vi "PolarizationSimulation.vi"() -> ()   [LabVIEW 2020]
uses:
  D:/LabVIEW/Integrated-Neural-Net-master/Integrated-Neural-Net-master (1)/Integrated-Neural-Net-master/Integrated ANN/Sub-VIs/Adam_data.ctl
  <vilib>/Utility/xml.llb/Read From XML File(string).vi
  <vilib>/Utility/xml.llb/Write to XML File(string).vi
  <vilib>/Analysis/NI_AALBase.lvlib
panel:
  in  "Regularization":T1
  in  "Batch Size":i16
  out "NN Loss":dbl(graph)
  in  "Loss Function":enum16{"MSE", "MAE"}(ring)
  in  "Parameters File Path":path
  out "NN Error":dbl
  in  "Training?":bool
  out "NN Output":dbl
  in  "Speed\nMultiplier":dbl=1.0
  in  "AFP On":bool
  in  "AFP Efficiency":dbl=0.9 min=0.0 max=1.0 step=0.01
  in  "AFP Control":cluster{i32, i32}(slide)={200, 230} scale=0.0..500.0
  out "lower R-value AFP":dbl
  out "upper R-value AFP":dbl
  in  "STOP":bool
  in  "Microwave Power":dbl=1.0
  in  "Lower Fit\nParameter":dbl=-3.6
  in  "Upper Fit\nParameter":dbl=3.6
  in  "Std Dev Noise":dbl step=0.0001
  out "lower R-value":dbl
  out "upper R-value":dbl
  in  "RF Control":cluster{i32, i32}(slide)={200, 230} scale=0.0..500.0
  out "p":dbl format="%_4g"
  out "r":dbl
  in  "Saturation\nPolarization":dbl=0.8 min=0.0 max=0.99 step=0.01
  out "Reimann \nsum of Q":dbl format="%_4g"
  out "Corrected Data (Q)":cluster{dbl[], dbl[]}(graph)
  in  "Select Target Type":u16(ring)=2 items=["Test Case", "Deuteron"]
  in  "Reset":bool
  out "Total Polarization (P)":cluster{dbl, dbl}(graph)
  in  "Spin Manipulation\nPower Factor":dbl=0.005
  in  "Decay Spin\nManipulation":bool
  out "Reimann\nsum of P":dbl format="%_4g"
  out "Corrected Data (P)":cluster{dbl[], dbl[]}[](graph)
  out "Signal and Fit (P)":cluster{dbl[], "Best Polynomial Fit":dbl[]}[](graph)
  in  "Positive\nPolarization":bool
  in  "Microwave on":bool
  # "Neural Network"
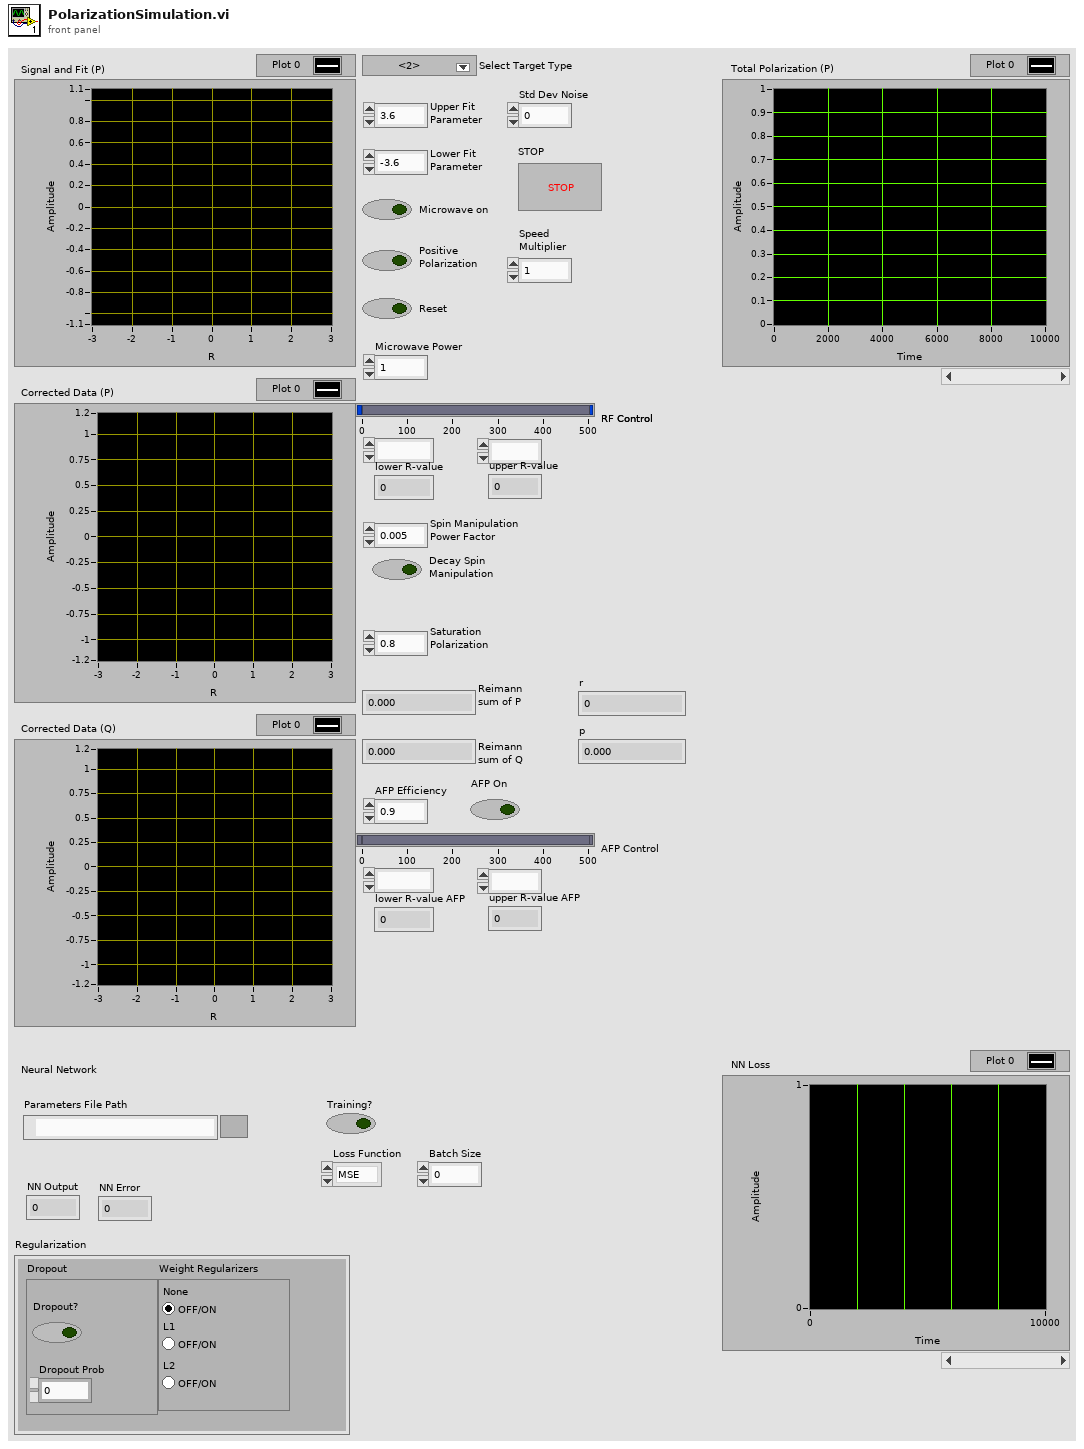
[diagram p1: front panel]
types:
  T1 = cluster{"Dropout":cluster{"Dropout?":bool, "Dropout Prob":dbl}, "Weight Regularizers":enum32{"None", "L1", "L2"}}
  T2 = typedef "Adam_data.ctl" = cluster{"Mw Moments":cluster{"3 ":dbl[], "2":dbl[][], "1":dbl[][]}, "Vw Moments":cluster{"3":dbl[], "2":dbl[][], "1":dbl[][]}, "Mb Moments":cluster{"3":dbl, "2":dbl[], "1":dbl[]}, "Vb Moments":cluster{"3":dbl, "2":dbl[], "1":dbl[]}}
  T3 = cluster{cluster{dbl[][], dbl[]}, cluster{dbl[][], dbl[]}, cluster{dbl[], dbl}}
  T4 = cluster{cluster{"Updated Weights":dbl[][], "Updated Biases":dbl[]}, cluster{"Updated Weights":dbl[][], "Updated Biases":dbl[]}, cluster{"Updated Weights":dbl[], "Updated Biases":dbl}}
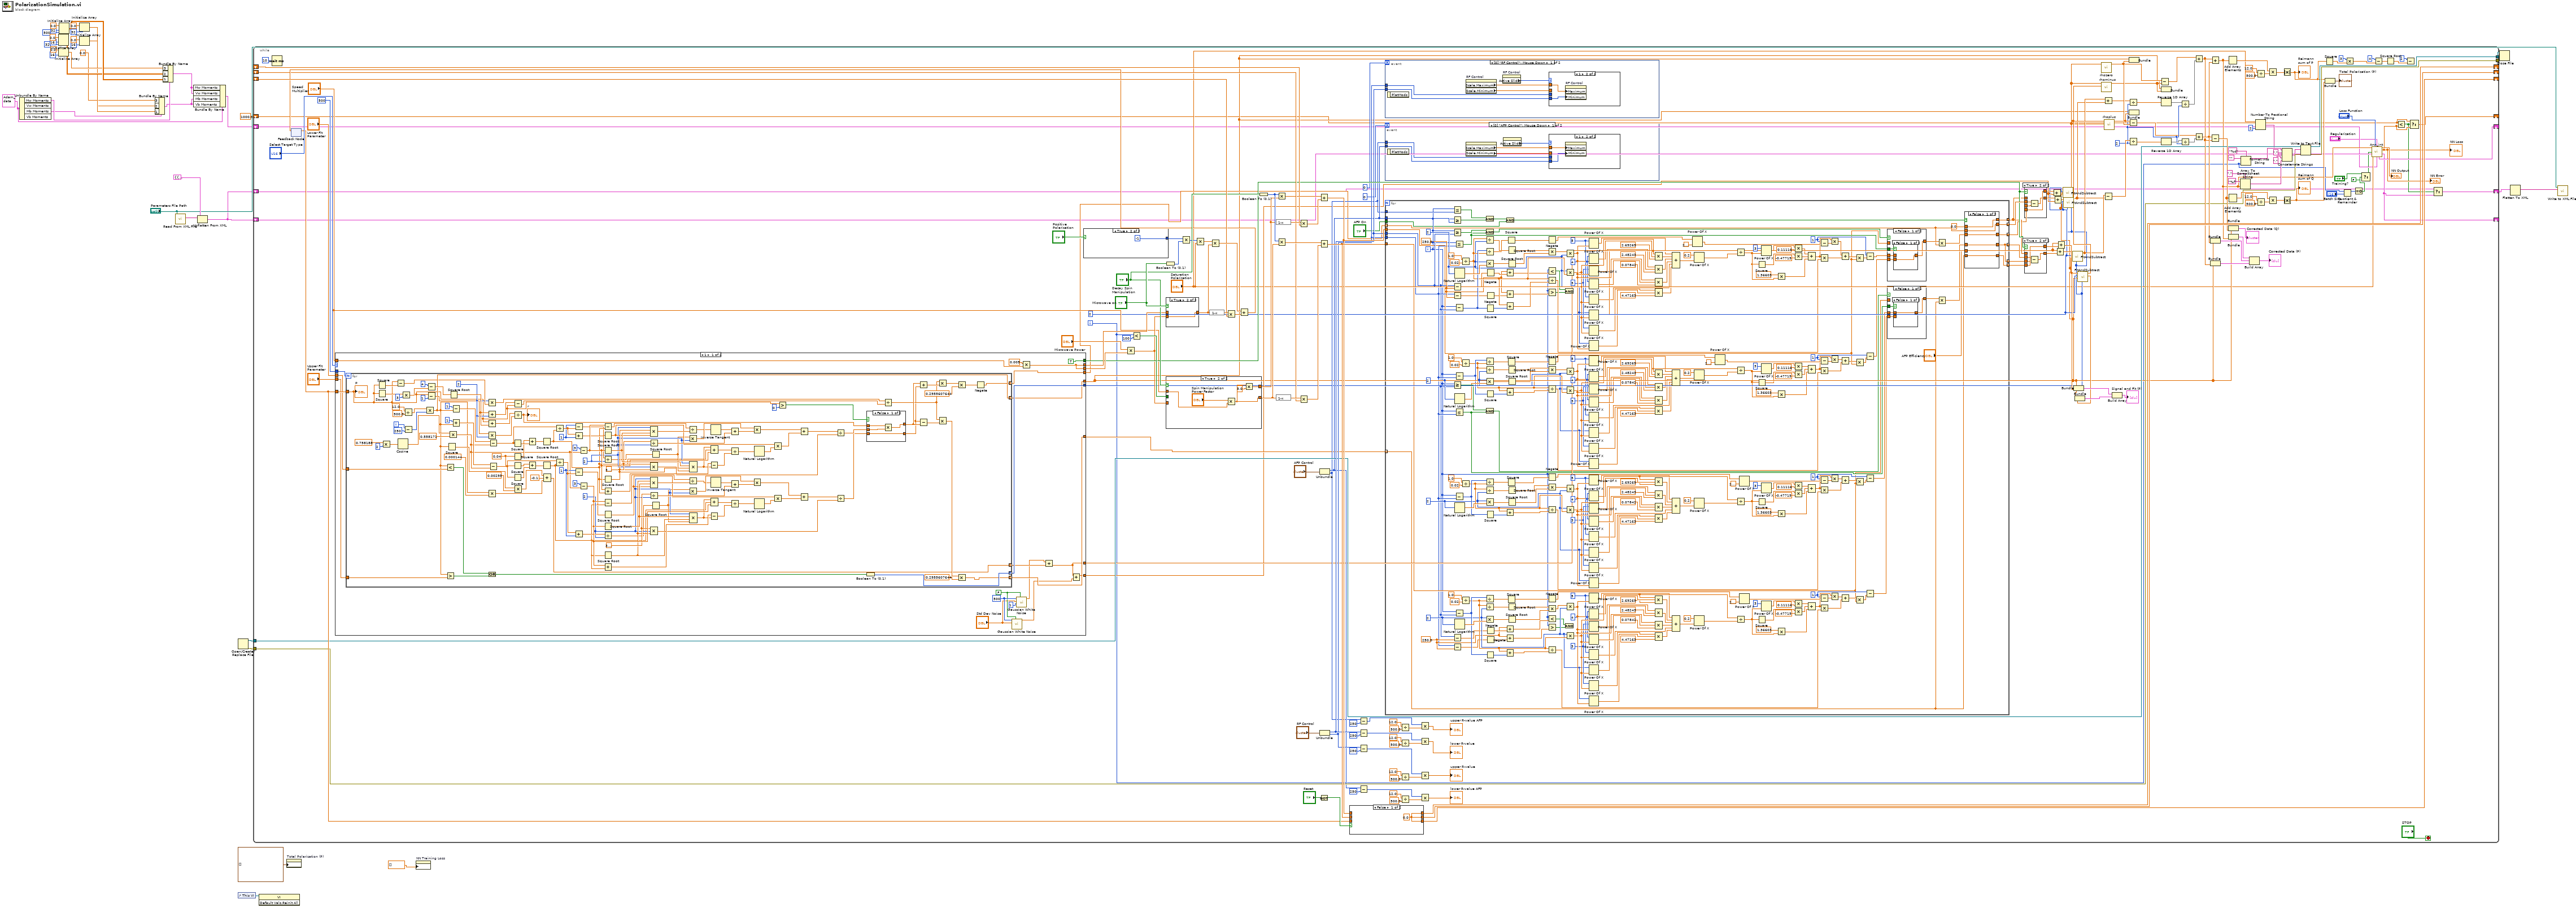
[diagram p0: block diagram]
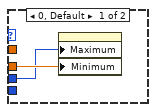
[diagram p2: hidden frame]
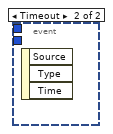
[diagram p3: hidden frame]
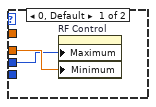
[diagram p4: hidden frame]
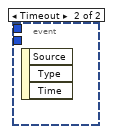
[diagram p5: hidden frame]
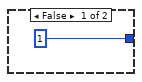
[diagram p6: hidden frame]
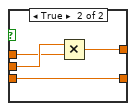
[diagram p7: hidden frame]
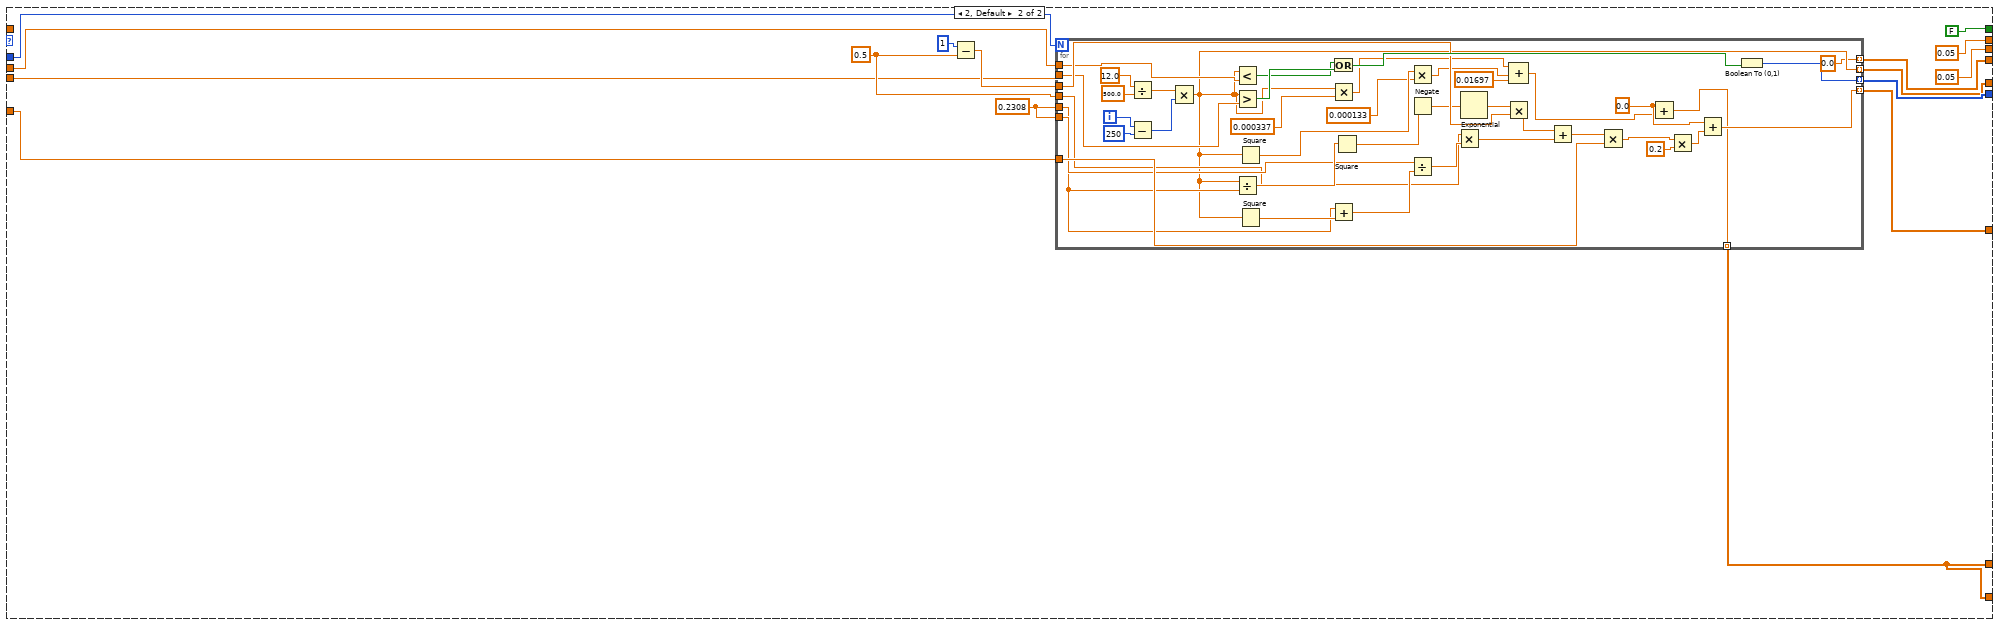
[diagram p8: hidden frame]
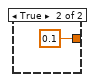
[diagram p10: hidden frame]
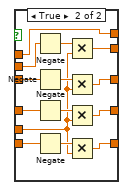
[diagram p15: hidden frame]
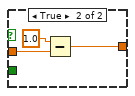
[diagram p17: hidden frame]
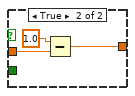
[diagram p19: hidden frame]
diagram:
  w7 = T2 {"Mw Moments"={"3 "=[], "2"=[], "1"=[]}, "Vw Moments"={"3"=[], "2"=[], "1"=[]}, "Mb Moments"={"3"=0.0, "2"=[], "1"=[]}, "Vb Moments"={"3"=0.0, "2"=[], "1"=[]}} ("Adam Data In")
  n1 = Unbundle By Name(w7) -> ("Mw Moments"=w9:cluster{"3 ":dbl[], "2":dbl[][], "1":dbl[][]}, "Mb Moments"=w8:cluster{"3":dbl, "2":dbl[], "1":dbl[]})  [unwired: 2 out]
  n2 = Initialize Array(0.0 ("element"), 16 ("dimension size"), 32 ("dimension size")) -> (w14:dbl[][])
  n3 = Initialize Array(0.0 ("element"), 16 ("dimension size")) -> (w13:dbl[])
  n4 = Initialize Array(0.0 ("element"), 32 ("dimension size"), 500 ("dimension size")) -> (w15:dbl[][])
  n5 = Initialize Array(0.0 ("element"), 16 ("dimension size")) -> (w11:dbl[])
  n6 = Initialize Array(0.0 ("element"), 32 ("dimension size")) -> (w12:dbl[])
  n7 = Bundle By Name(cluster=w8, "3"=0.0 ("element"), "2"=w11, "1"=w12) -> (w5:cluster{"3":dbl, "2":dbl[], "1":dbl[]})
  n8 = Bundle By Name(cluster=w9, "3"=w13, "2"=w14, "1"=w15) -> (w6:cluster{"3 ":dbl[], "2":dbl[][], "1":dbl[][]})
  n9 = call-poly <vilib>:"Read From XML File.vi"("XML File Path"="Parameters File Path") -> ("XML Elements"=w32:string)  [unwired: 8 in, 2 out]
  n10 = Bundle By Name(cluster=w7, "Mw Moments"=w6, "Vw Moments"=w6, "Mb Moments"=w5, "Vb Moments"=w5) -> (w4:T2)
  n11 = Unflatten From XML(xml string=w32, type=T3 {{[], []}, {[], []}, {[], 0.0}}) -> (value=w3:T3)  [unwired: 1 in, 1 out]
  n12 = Open/Create/Replace File() -> (refnum out=w36:refnum<file>, error out=w35:errorcluster)  [unwired: 6 in, 1 out]
  n13 = control-ref of="This VI"() -> (w38:refnum<vi>)
  n14 = while {
    shift-right: [w212] -> _
    shift-left: _ -> [w219]
    shift-right: [w211] -> _
    shift-left: _ -> [w194]
    shift-right: [w189] -> _
    shift-left: _ -> [w188]
    tunnel: w36 -> [w121]
    tunnel: w35 -> [w120]
    tunnel: [w119] -> w34
    tunnel: [w118] -> w33
    shift-right: [w42] -> _
    shift-left: w3 -> [w58]
    shift-right: [w55] -> _
    shift-left: w4 -> [w54]
    shift-right: [w46] -> _
    shift-left: 1000.0 ("Error") -> [w45]
    shift-right: [w41] -> w2
    shift-left: w3 -> [w40]
    i -> [w53]
    stop <- "STOP" stop-if-true
    w171 = 2
    w67 = 2
    n15 = Wait (ms)(milliseconds to wait=10) -> ()  [unwired: 1 out]
    n16 = feedback #1() -> (w198:dbl)  [unwired: 1 in]
    n17 = case shown="1" "Select Target Type" {
      tunnel: [w254 0.05 ("Growth Constant")] -> w203
      tunnel: [w254 0.05 ("Decay Constant")] -> w202
      tunnel: 500 -> [w263 w421]
      tunnel: w198 -> [w266 w420]
      tunnel: "Upper Fit\nParameter" -> [w264 w418]
      tunnel: "Lower Fit\nParameter" -> [w265 w419]
      tunnel: [w261 w416] -> w66
      tunnel: [w251 w415] -> w81
      tunnel: [w262 w417] -> w65
      tunnel: [TRUE FALSE] -> w182
      tunnel: [w252 w411] -> w80
      tunnel: "Speed\nMultiplier" -> [w253 _]
      tunnel: [w247 w410] -> w79
      tunnel: [w249 w410] -> w78
      frame 1 {
        w256 = FALSE
        w258 = 500
        n18 = for {
          N: w263 -> [_]
          tunnel: [w297] -> w261 mode=indexing
          tunnel: [w386] -> w262 mode=indexing
          tunnel: w264 -> [w385]
          tunnel: w265 -> [w384]
          tunnel: [w269] -> w251 mode=indexing
          tunnel: w266 -> [w270]
          tunnel: [w268] -> w252 mode=indexing
          tunnel: [w267] -> w250 mode=indexing
          i -> [w362]
          w284 = 2
          w323 = 1
          w327 = 3.141592653589793
          w321 = 2
          w306 = 0.04
          w359 = 1
          w364 = 3.141592653589793
          w357 = 2
          n19 = Square(x=w270) -> (x^2=w287:dbl)
          n20 = Square(x=w270) -> (x^2=w313:dbl)
          n21 = Multiply(x=0.758188, y=2) -> (x*y=w301:dbl)
          n22 = Subtract(x=w270, y=w287) -> (x-y=w286:dbl)
          n23 = Cosine(x=w301) -> (cos(x)=w304:dbl)
          n24 = Multiply(x=w313, y=3) -> (x*y=w312:dbl)
          n25 = Divide(x=12.0, y=500.0) -> (x/y=w400:dbl)
          n26 = Subtract(x=w362, y=250) -> (x-y=w399:i32)
          n27 = Multiply(x=w400, y=w399) -> (x*y=w297:dbl)
          n28 = Subtract(x=4, y=w312) -> (x-y=w310:dbl)
          n29 = Subtract(x=w270, y=1) -> (x-y=w308:dbl)
          n30 = Less?(x=w297, y=w384) -> (x < y?=w389:bool)
          n31 = Greater?(x=w297, y=w385) -> (0:w388:bool)
          n32 = Square(x=w297) -> (x^2=w299:dbl)
          n33 = Multiply(x=w304, y=0.558171) -> (x*y=w305:dbl)
          n34 = Square Root(x=w310) -> (sqrt(x)=w285:dbl)
          n35 = Subtract(x=1, y=w297) -> (x-y=w394:dbl)
          n36 = Add(x=1, y=w297) -> (x+y=w351:dbl)
          n37 = Multiply(x=w284, y=w286) -> (x*y=w282:dbl)
          n38 = Add(x=w285, y=w284) -> (x+y=w283:dbl)
          n39 = Add(x=w270, y=w285) -> (x+y=w309:dbl)
          n40 = Multiply(x=w308, y=w284) -> (x*y=w292:dbl)
          n41 = Multiply(x=w297, y=0.000144) -> (x*y=w294:dbl)
          n42 = Or(x=w389, y=w388) -> (x .or. y?=w387:bool)
          n43 = Subtract(x=w394, y=w305) -> (x-y=w390:dbl)
          n44 = Subtract(x=w351, y=w305) -> (x-y=w347:dbl)
          n45 = Square(x=w390) -> (x^2=w393:dbl)
          n46 = Square(x=w306) -> (x^2=w392:dbl)
          n47 = Square(x=w306) -> (x^2=w349:dbl)
          n48 = Square(x=w347) -> (x^2=w350:dbl)
          n49 = Subtract(x=w283, y=w270) -> (x-y=w281:dbl)
          n50 = Divide(x=w309, y=w292) -> (x/y=w288:dbl)
          "r" <- w288
          n51 = Multiply(x=w299, y=0.00295) -> (x*y=w298:dbl)
          n52 = Add(x=w392, y=w393) -> (x+y=w391:dbl)
          n53 = Add(x=w349, y=w350) -> (x+y=w348:dbl)
          n54 = Square Root(x=w391) -> (sqrt(x)=w354:dbl)
          n55 = Square Root(x=w348) -> (sqrt(x)=w318:dbl)
          n56 = Compound Arithmetic op=ADD(w298, -0.1, w294) -> (w267:dbl)
          n57 = Divide(x=w390, y=w354) -> (x/y=w360:dbl)
          n58 = Divide(x=w347, y=w318) -> (x/y=w324:dbl)
          n59 = Subtract(x=w359, y=w360) -> (x-y=w315:dbl)
          n60 = Add(x=w360, y=w359) -> (x+y=w358:dbl)
          n61 = Subtract(x=w323, y=w324) -> (x-y=w316:dbl)
          n62 = Add(x=w324, y=w323) -> (x+y=w322:dbl)
          n63 = Subtract(x=3, y=w305) -> (x-y=w370:dbl)
          n64 = Subtract(x=3, y=w305) -> (x-y=w333:dbl)
          n65 = Subtract(x=w370, y=w354) -> (x-y=w379:dbl)
          n66 = Square Root(x=w315) -> (sqrt(x)=w361:dbl)
          n67 = Square Root(x=w370) -> (sqrt(x)=w373:dbl)
          n68 = Divide(x=w358, y=w357) -> (x/y=w356:dbl)
          n69 = Square Root(x=w354) -> (sqrt(x)=w363:dbl)
          n70 = Add(x=w370, y=w354) -> (x+y=w369:dbl)
          n71 = Subtract(x=w333, y=w318) -> (x-y=w342:dbl)
          n72 = Square Root(x=w316) -> (sqrt(x)=w325:dbl)
          n73 = Square Root(x=w333) -> (sqrt(x)=w336:dbl)
          n74 = Divide(x=w322, y=w321) -> (x/y=w320:dbl)
          n75 = Square Root(x=w318) -> (sqrt(x)=w326:dbl)
          n76 = Add(x=w333, y=w318) -> (x+y=w332:dbl)
          n77 = Divide(x=w364, y=w357) -> (x/y=w381:dbl)
          n78 = Divide(x=w327, y=w321) -> (x/y=w344:dbl)
          n79 = Compound Arithmetic op=MULTIPLY(w357, w363, w373, w361) -> (w378:dbl)
          n80 = Compound Arithmetic op=MULTIPLY(w364, w357, w363) -> (w365:dbl)
          n81 = Compound Arithmetic op=MULTIPLY(w321, w326, w336, w325) -> (w341:dbl)
          n82 = Compound Arithmetic op=MULTIPLY(w327, w321, w326) -> (w328:dbl)
          n83 = Square Root(x=w356) -> (sqrt(x)=w355:dbl)
          n84 = Square Root(x=w320) -> (sqrt(x)=w319:dbl)
          n85 = Divide(x=w379, y=w378) -> (x/y=w377:dbl)
          n86 = Multiply(x=w355, y=w357) -> (x*y=w383:dbl)
          n87 = Divide(x=w342, y=w341) -> (x/y=w340:dbl)
          n88 = Multiply(x=w319, y=w321) -> (x*y=w346:dbl)
          n89 = Compound Arithmetic op=MULTIPLY(w357, w373, w363, w355) -> (w368:dbl)
          n90 = Compound Arithmetic op=MULTIPLY(w321, w336, w326, w319) -> (w331:dbl)
          n91 = Subtract(x=w369, y=w368) -> (x-y=w367:dbl)
          n92 = Subtract(x=w332, y=w331) -> (x-y=w330:dbl)
          n93 = Inverse Tangent(1:w377) -> (0:w382:dbl)
          n94 = Compound Arithmetic op=ADD(w368, w354, w370) -> (w372:dbl)
          n95 = Inverse Tangent(1:w340) -> (0:w345:dbl)
          n96 = Compound Arithmetic op=ADD(w331, w318, w333) -> (w335:dbl)
          n97 = Add(x=w382, y=w381) -> (x+y=w380:dbl)
          n98 = Divide(x=w372, y=w367) -> (x/y=w371:dbl)
          n99 = Add(x=w345, y=w344) -> (x+y=w343:dbl)
          n100 = Divide(x=w335, y=w330) -> (x/y=w334:dbl)
          n101 = Multiply(x=w383, y=w380) -> (x*y=w376:dbl)
          n102 = Multiply(x=w346, y=w343) -> (x*y=w339:dbl)
          n103 = Natural Logarithm(1:w371) -> (0:w374:dbl)
          n104 = Natural Logarithm(1:w334) -> (0:w337:dbl)
          n105 = Multiply(x=w361, y=w374) -> (x*y=w375:dbl)
          n106 = Multiply(x=w325, y=w337) -> (x*y=w338:dbl)
          n107 = Greater?(x=w270, y=0) -> (0:w272:bool)
          n108 = Add(x=w376, y=w375) -> (x+y=w366:dbl)
          n109 = Add(x=w339, y=w338) -> (x+y=w329:dbl)
          n110 = Divide(x=w366, y=w365) -> (x/y=w307:dbl)
          n111 = Divide(x=w329, y=w328) -> (x/y=w274:dbl)
          n112 = Boolean To (0,1)(Boolean=w387) -> (0, 1=w386:i16)
          n113 = case shown="False" w272 {
            tunnel: w307 -> [w404 w409]
            tunnel: [w402 w408] -> w290
            tunnel: w288 -> [w405 w407]
            tunnel: w274 -> [w403 w406]
            tunnel: [w403 w406] -> w273
            frame False {
              n114 = Multiply(x=w405, y=w404) -> (x*y=w402:dbl)
            }
            frame True {
              n115 = Multiply(x=w409, y=w407) -> (x*y=w408:dbl)
            }
          }
          n116 = Divide(x=w282, y=w281) -> (x/y=w280:dbl)
          n117 = Add(x=w290, y=w273) -> (x+y=w291:dbl)
          n118 = Subtract(x=w273, y=w290) -> (x-y=w317:dbl)
          n119 = Multiply(x=w280, y=w291) -> (x*y=w279:dbl)
          n120 = Multiply(x=w280, y=w317) -> (x*y=w278:dbl)
          n121 = Multiply(x=w279, y=0.2955607644) -> (x*y=w277:dbl)
          n122 = Multiply(x=w278, y=0.2955607644) -> (x*y=w269:dbl)
          n123 = Negate(x=w277) -> (-x=w268:dbl)
          "p" <- w270
        }
        n124 = call <vilib>:"Gaussian White Noise.vi"("initialize?"=w256, "standard deviation"="Std Dev Noise", "samples"=w258) -> ("Gaussian noise pattern"=w248:dbl[])  [unwired: 7 in, 1 out]
        n125 = call <vilib>:"Gaussian White Noise.vi"("initialize?"=w256, "seed"=1, "standard deviation"="Std Dev Noise", "samples"=w258) -> ("Gaussian noise pattern"=w246:dbl[])  [unwired: 6 in, 1 out]
        n126 = Multiply(x=0.005, y=w253) -> (x*y=w254:dbl)
        n127 = Add(x=w246, y=w250) -> (x+y=w247:dbl[])
        n128 = Add(x=w247, y=w248) -> (x+y=w249:dbl[])
      }
      frame 2, Default {
        w422 = 0.2308
        w423 = 0.5
        n129 = Subtract(x=1, y=w423) -> (x-y=w425:dbl)
        n130 = for {
          N: w421 -> [_]
          tunnel: w420 -> [w465]
          tunnel: [w431] -> w416 mode=indexing
          tunnel: [w449] -> w415 mode=indexing
          tunnel: [w463] -> w417 mode=indexing
          tunnel: w425 -> [w459]
          tunnel: w422 -> [w457]
          tunnel: w422 -> [w438]
          tunnel: w423 -> [w451]
          tunnel: w418 -> [w446]
          tunnel: w419 -> [w445]
          tunnel: [0.0] -> w411 mode=indexing
          tunnel: [w426] -> w410 mode=indexing
          i -> [w439]
          w450 = 0.0
          n131 = Divide(x=12.0, y=500.0) -> (x/y=w440:dbl)
          n132 = Subtract(x=w439, y=250) -> (x-y=w444:i32)
          n133 = Multiply(x=w440, y=w444) -> (x*y=w431:dbl)
          n134 = Less?(x=w431, y=w445) -> (x < y?=w460:bool)
          n135 = Greater?(x=w431, y=w446) -> (0:w461:bool)
          n136 = Divide(x=w431, y=w438) -> (x/y=w466:dbl)
          n137 = Square(x=w431) -> (x^2=w434:dbl)
          n138 = Square(x=w431) -> (x^2=w456:dbl)
          n139 = Or(x=w460, y=w461) -> (x .or. y?=w462:bool)
          n140 = Multiply(x=w431, y=0.000337) -> (x*y=w433:dbl)
          n141 = Add(x=w438, y=w456) -> (x+y=w458:dbl)
          n142 = Square(x=w466) -> (x^2=w467:dbl)
          n143 = Multiply(x=w434, y=0.000133) -> (x*y=w432:dbl)
          n144 = Negate(x=w467) -> (-x=w448:dbl)
          n145 = Divide(x=w457, y=w458) -> (x/y=w453:dbl)
          n146 = Multiply(x=w451, y=w453) -> (x*y=w452:dbl)
          n147 = Exponential(1:w448) -> (0:w447:dbl)
          n148 = Multiply(x=w447, y=w459) -> (x*y=w455:dbl)
          n149 = Compound Arithmetic op=ADD(w433, w432, 0.01697) -> (w435:dbl)
          n150 = Add(x=w455, y=w452) -> (x+y=w454:dbl)
          n151 = Multiply(x=w454, y=w465) -> (x*y=w464:dbl)
          n152 = Add(x=w450, y=w435) -> (x+y=w426:dbl)
          n153 = Multiply(x=w464, y=0.2) -> (x*y=w437:dbl)
          n154 = Add(x=w450, y=w437) -> (x+y=w449:dbl)
          n155 = Boolean To (0,1)(Boolean=w462) -> (0, 1=w463:i16)
        }
      }
    }
    n156 = case shown="True" "Positive\nPolarization" {
      tunnel: [1 -1] -> w156
      frame False {
      }
      frame True {
      }
    }
    n157 = Multiply(x="Microwave Power", y=w203) -> (x*y=w124:dbl)
    n158 = Less?(x=w53, y=100) -> (x < y?=w214:bool)
    n159 = Boolean To (0,1)(Boolean="Microwave on") -> (0, 1=w221:i16)
    n160 = case shown="True" "Microwave on" {
      tunnel: [w478 w479] -> w206
      tunnel: w124 -> [_ w479]
      tunnel: w202 -> [w478 _]
      frame False {
      }
      frame True {
      }
    }
    n161 = case shown="True" "Decay Spin\nManipulation" {
      tunnel: [w468 w474] -> w215
      tunnel: w124 -> [w470 _]
      tunnel: w214 -> [w469 _]
      tunnel: [w468 w475] -> w196
      tunnel: "Speed\nMultiplier" -> [_ w473]
      frame False {
        n162 = case shown="False" w469 {
          tunnel: [w471 0.1] -> w468
          tunnel: w470 -> [w471 _]
          frame False {
          }
          frame True {
          }
        }
      }
      frame True {
        n163 = Multiply(x="Spin Manipulation\nPower Factor", y=w473) -> (x*y=w474:dbl)
        n164 = Multiply(x=w474, y=3.0) -> (x*y=w475:dbl)
      }
    }
    n165 = Multiply(x=w156, y=w221) -> (x*y=w157:i32)
    n166 = Multiply(x=w157, y="Saturation\nPolarization") -> (x*y=w164:dbl)
    n167 = expression code="1-x"(w206) -> (w222:dbl)
    n168 = Multiply(x=w164, y=w206) -> (x*y=w223:dbl)
    n169 = Multiply(x=w222, y=w219) -> (x*y=w224:dbl)
    n170 = Add(x=w223, y=w224) -> (x+y=w201:dbl)
    n171 = feedback-in #1(w201) -> ()
    n172 = Boolean To (0,1)(Boolean="Decay Spin\nManipulation") -> (0, 1=w197:i16)
    n173 = expression code="1-x"(w196) -> (w195:dbl)
    n174 = expression code="1-x"(w215) -> (w216:dbl)
    n175 = Multiply(x=w197, y=w196) -> (x*y=w192:dbl)
    n176 = Multiply(x=w197, y=w215) -> (x*y=w217:dbl)
    n177 = Multiply(x=w195, y=w188) -> (x*y=w193:dbl)
    n178 = Multiply(x=w216, y=w194) -> (x*y=w218:dbl)
    n179 = Add(x=w192, y=w193) -> (x+y=w190:dbl)
    n180 = Add(x=w217, y=w218) -> (x+y=w210:dbl)
    n181 = Not(x="Reset") -> (.not. x?=w209:bool)
    n182 = Unbundle("AFP Control") -> (w88:i32, w87:i32)
    n183 = Unbundle("RF Control") -> (w127:i32, w126:i32)
    n184 = case shown="False" w209 {
      tunnel: [w492 w495] -> w212
      tunnel: w198 -> [_ w495]
      tunnel: [w492 w494] -> w211
      tunnel: w210 -> [_ w494]
      tunnel: w190 -> [_ w493]
      tunnel: [w492 w493] -> w189
      frame False {
        w492 = 0.0
      }
      frame True {
      }
    }
    n185 = Subtract(x=w87, y=250) -> (x-y=w94:i32)
    n186 = Subtract(x=w127, y=250) -> (x-y=w133:i32)
    n187 = Subtract(x=w126, y=250) -> (x-y=w136:i32)
    n188 = Subtract(x=w88, y=250) -> (x-y=w91:i32)
    n189 = event shown="[0] \"RF Control\": Mouse Down" {
      selector: _ -> [_ _]
      dyn-events: _ -> [_ _]
      timeout: 0 -> [_ _]
      tunnel: w127 -> [w236 _]
      tunnel: w126 -> [w235 _]
      event "RF Control": Mouse Down {
        n190 = event-data() -> ()  [unwired: 1 in, 1 out]
        n191 = property on="RF Control" class="Slide (strict)"() -> ("Scale.Maximum"=w237:dbl, "Scale.Minimum"=w238:dbl)  [unwired: 2 in, 2 out]
        n192 = property on="RF Control" class="Slide (strict)"() -> ("Active Slider"=w239:i32)  [unwired: 2 in, 2 out]
        n193 = case shown="1" w239 {
          tunnel: w238 -> [w241 _]
          tunnel: w235 -> [w240 _]
          tunnel: w237 -> [_ w243]
          tunnel: w236 -> [_ w242]
          frame 0, Default {
            n194 = property on="RF Control" class="Slide (strict)"("Maximum"=w240, "Minimum"=w241) -> ()  [unwired: 2 in, 2 out]
          }
          frame 1 {
            n195 = property on="RF Control" class="Slide (strict)"("Maximum"=w243, "Minimum"=w242) -> ()  [unwired: 2 in, 2 out]
          }
        }
      }
      event Timeout {
        n196 = event-data() -> ()  [unwired: 1 in, 3 out]
      }
    }
    n197 = event shown="[0] \"AFP Control\": Mouse Down" {
      selector: _ -> [_ _]
      dyn-events: _ -> [_ _]
      timeout: 0 -> [_ _]
      tunnel: w88 -> [w227 _]
      tunnel: w87 -> [w226 _]
      event "AFP Control": Mouse Down {
        n198 = event-data() -> ()  [unwired: 1 in, 1 out]
        n199 = property on="AFP Control" class="Slide (strict)"() -> ("Scale.Maximum"=w228:dbl, "Scale.Minimum"=w229:dbl)  [unwired: 2 in, 2 out]
        n200 = property on="AFP Control" class="Slide (strict)"() -> ("Active Slider"=w230:i32)  [unwired: 2 in, 2 out]
        n201 = case shown="1" w230 {
          tunnel: w229 -> [w232 _]
          tunnel: w226 -> [w231 _]
          tunnel: w228 -> [_ w234]
          tunnel: w227 -> [_ w233]
          frame 0, Default {
            n202 = property on="AFP Control" class="Slide (strict)"("Maximum"=w231, "Minimum"=w232) -> ()  [unwired: 2 in, 2 out]
          }
          frame 1 {
            n203 = property on="AFP Control" class="Slide (strict)"("Maximum"=w234, "Minimum"=w233) -> ()  [unwired: 2 in, 2 out]
          }
        }
      }
      event Timeout {
        n204 = event-data() -> ()  [unwired: 1 in, 3 out]
      }
    }
    n205 = for {
      tunnel: w81 -> [w508] mode=indexing
      tunnel: w210 -> [w660]
      tunnel: w126 -> [w518]
      tunnel: w127 -> [w517]
      tunnel: [w504] -> w200 mode=indexing
      tunnel: [w505] -> w191 mode=indexing
      tunnel: [w505] -> w199 mode=indexing
      tunnel: w80 -> [w497] mode=indexing
      tunnel: w190 -> [w516]
      tunnel: [w496] -> w186 mode=indexing
      tunnel: [w503] -> w176 mode=indexing
      tunnel: w88 -> [w512]
      tunnel: w87 -> [w511]
      tunnel: "AFP On" -> [w500]
      tunnel: [w499] -> w85 mode=indexing
      i -> [w510]
      w520 = 250.0
      w559 = 5
      w557 = 4
      w556 = 3
      w537 = 1
      w538 = 2
      w620 = 5
      w618 = 4
      w617 = 3
      w597 = 1
      w598 = 2
      w654 = 250.0
      w695 = 5
      w693 = 4
      w692 = 3
      w673 = 1
      w674 = 2
      w756 = 5
      w754 = 4
      w753 = 3
      w733 = 1
      w734 = 2
      n206 = Less Or Equal?(x=w510, y=w511) -> (x <= y?=w513:bool)
      n207 = Greater Or Equal?(x=w510, y=w512) -> (x >= y?=w514:bool)
      n208 = Greater Or Equal?(x=w510, y=w517) -> (x >= y?=w593:bool)
      n209 = Subtract(x=w517, y=w520) -> (x-y=w524:dbl)
      n210 = Subtract(x=w518, y=w520) -> (x-y=w525:dbl)
      n211 = Greater Or Equal?(x=w510, y=w517) -> (x >= y?=w729:bool)
      n212 = Subtract(x=w517, y=w654) -> (x-y=w658:dbl)
      n213 = Subtract(x=w518, y=w654) -> (x-y=w659:dbl)
      n214 = Less Or Equal?(x=w510, y=w518) -> (x <= y?=w530:bool)
      n215 = Natural Logarithm(1:w598) -> (0:w633:dbl)
      n216 = Subtract(x=w510, y=w517) -> (x-y=w606:i32)
      n217 = Subtract(x=w510, y=w518) -> (x-y=w545:i32)
      n218 = Natural Logarithm(1:w538) -> (0:w572:dbl)
      n219 = Less Or Equal?(x=w510, y=w518) -> (x <= y?=w665:bool)
      n220 = Subtract(x=w510, y=w518) -> (x-y=w681:i32)
      n221 = Natural Logarithm(1:w674) -> (0:w708:dbl)
      n222 = Subtract(x=w510, y=w517) -> (x-y=w742:i32)
      n223 = Natural Logarithm(1:w734) -> (0:w769:dbl)
      n224 = Divide(x=1.0, y=0.02) -> (x/y=w602:dbl)
      n225 = Divide(x=1.0, y=0.02) -> (x/y=w542:dbl)
      n226 = Divide(x=1.0, y=0.02) -> (x/y=w678:dbl)
      n227 = Divide(x=1.0, y=0.02) -> (x/y=w738:dbl)
      n228 = And(x=w513, y=w514) -> (x .and. y?=w502:bool)
      n229 = And(x=w593, y=w530) -> (x .and. y?=w531:bool)
      n230 = Divide(x=w602, y=w598) -> (x/y=w631:dbl)
      n231 = Divide(x=w606, y=w602) -> (x/y=w610:dbl)
      n232 = Multiply(x=w598, y=w633) -> (x*y=w634:dbl)
      n233 = Divide(x=w545, y=w542) -> (x/y=w549:dbl)
      n234 = Divide(x=w542, y=w538) -> (x/y=w570:dbl)
      n235 = Multiply(x=w538, y=w572) -> (x*y=w573:dbl)
      n236 = And(x=w729, y=w665) -> (x .and. y?=w667:bool)
      n237 = Divide(x=w681, y=w678) -> (x/y=w685:dbl)
      n238 = Divide(x=w678, y=w674) -> (x/y=w706:dbl)
      n239 = Multiply(x=w674, y=w708) -> (x*y=w709:dbl)
      n240 = Divide(x=w742, y=w738) -> (x/y=w746:dbl)
      n241 = Divide(x=w738, y=w734) -> (x/y=w767:dbl)
      n242 = Multiply(x=w734, y=w769) -> (x*y=w770:dbl)
      n243 = Square(x=w606) -> (x^2=w607:i32)
      n244 = Square(x=w545) -> (x^2=w546:i32)
      n245 = Square(x=w681) -> (x^2=w682:i32)
      n246 = Square(x=w742) -> (x^2=w743:i32)
      n247 = Negate(x=w524) -> (-x=w523:dbl)
      n248 = Negate(x=w525) -> (-x=w521:dbl)
      n249 = Negate(x=w658) -> (-x=w657:dbl)
      n250 = Negate(x=w659) -> (-x=w655:dbl)
      n251 = Add(x=w520, y=w523) -> (x+y=w522:dbl)
      n252 = Add(x=w520, y=w521) -> (x+y=w519:dbl)
      n253 = Add(x=w602, y=w607) -> (x+y=w608:dbl)
      n254 = Add(x=w542, y=w546) -> (x+y=w547:dbl)
      n255 = Add(x=w678, y=w682) -> (x+y=w683:dbl)
      n256 = Add(x=w654, y=w657) -> (x+y=w656:dbl)
      n257 = Add(x=w654, y=w655) -> (x+y=w653:dbl)
      n258 = Add(x=w738, y=w743) -> (x+y=w744:dbl)
      n259 = And(x=w502, y=w500) -> (x .and. y?=w501:bool)
      n260 = Square(x=w610) -> (x^2=w612:dbl)
      n261 = Square(x=w549) -> (x^2=w551:dbl)
      n262 = Square(x=w685) -> (x^2=w687:dbl)
      n263 = Square(x=w746) -> (x^2=w748:dbl)
      n264 = Square Root(x=w631) -> (sqrt(x)=w632:dbl)
      n265 = Square Root(x=w634) -> (sqrt(x)=w635:dbl)
      n266 = Square Root(x=w570) -> (sqrt(x)=w571:dbl)
      n267 = Square Root(x=w573) -> (sqrt(x)=w574:dbl)
      n268 = Square Root(x=w706) -> (sqrt(x)=w707:dbl)
      n269 = Square Root(x=w709) -> (sqrt(x)=w710:dbl)
      n270 = Square Root(x=w767) -> (sqrt(x)=w768:dbl)
      n271 = Square Root(x=w770) -> (sqrt(x)=w771:dbl)
      n272 = Negate(x=w612) -> (-x=w611:dbl)
      n273 = Multiply(x=w632, y=w635) -> (x*y=w626:dbl)
      n274 = Less?(x=w510, y=w522) -> (x < y?=w527:bool)
      n275 = Divide(x=w602, y=w608) -> (x/y=w605:dbl)
      n276 = Greater?(x=w510, y=w519) -> (0:w526:bool)
      n277 = Negate(x=w551) -> (-x=w550:dbl)
      n278 = Multiply(x=w571, y=w574) -> (x*y=w565:dbl)
      n279 = Divide(x=w542, y=w547) -> (x/y=w532:dbl)
      n280 = Negate(x=w687) -> (-x=w686:dbl)
      n281 = Multiply(x=w707, y=w710) -> (x*y=w701:dbl)
      n282 = Divide(x=w678, y=w683) -> (x/y=w668:dbl)
      n283 = Negate(x=w748) -> (-x=w747:dbl)
      n284 = Multiply(x=w768, y=w771) -> (x*y=w762:dbl)
      n285 = Less?(x=w510, y=w656) -> (x < y?=w662:bool)
      n286 = Greater?(x=w510, y=w653) -> (0:w661:bool)
      n287 = Divide(x=w738, y=w744) -> (x/y=w741:dbl)
      n288 = And(x=w527, y=w526) -> ()  [unwired: 1 out]
      n289 = And(x=w662, y=w661) -> ()  [unwired: 1 out]
      n290 = Multiply(x=w626, y=w598) -> (x*y=w650:dbl)
      n291 = Multiply(x=w598, y=w602) -> (x*y=w644:dbl)
      n292 = Multiply(x=w565, y=w538) -> (x*y=w589:dbl)
      n293 = Multiply(x=w538, y=w542) -> (x*y=w583:dbl)
      n294 = Multiply(x=w701, y=w674) -> (x*y=w725:dbl)
      n295 = Multiply(x=w674, y=w678) -> (x*y=w719:dbl)
      n296 = Multiply(x=w762, y=w734) -> (x*y=w786:dbl)
      n297 = Multiply(x=w734, y=w738) -> (x*y=w780:dbl)
      n298 = Power Of X(1:w650, 2:w620) -> (0:w637:dbl)
      n299 = Power Of X(1:w650, 2:w618) -> (0:w643:dbl)
      n300 = Power Of X(1:w650, 2:w617) -> (0:w645:dbl)
      n301 = Power Of X(1:w644, 2:w618) -> (0:w649:dbl)
      n302 = Power Of X(1:w644, 2:w620) -> (0:w638:dbl)
      n303 = Power Of X(1:w644, 2:w598) -> (0:w646:dbl)
      n304 = Power Of X(1:w644, 2:w617) -> (0:w647:dbl)
      n305 = Power Of X(1:w650, 2:w598) -> (0:w648:dbl)
      n306 = Power Of X(1:w589, 2:w559) -> (0:w576:dbl)
      n307 = Power Of X(1:w589, 2:w557) -> (0:w582:dbl)
      n308 = Power Of X(1:w589, 2:w556) -> (0:w584:dbl)
      n309 = Power Of X(1:w583, 2:w557) -> (0:w588:dbl)
      n310 = Power Of X(1:w583, 2:w559) -> (0:w577:dbl)
      n311 = Power Of X(1:w583, 2:w538) -> (0:w585:dbl)
      n312 = Power Of X(1:w583, 2:w556) -> (0:w586:dbl)
      n313 = Power Of X(1:w589, 2:w538) -> (0:w587:dbl)
      n314 = Power Of X(1:w725, 2:w695) -> (0:w712:dbl)
      n315 = Power Of X(1:w725, 2:w693) -> (0:w718:dbl)
      n316 = Power Of X(1:w725, 2:w692) -> (0:w720:dbl)
      n317 = Power Of X(1:w719, 2:w693) -> (0:w724:dbl)
      n318 = Power Of X(1:w719, 2:w695) -> (0:w713:dbl)
      n319 = Power Of X(1:w719, 2:w674) -> (0:w721:dbl)
      n320 = Power Of X(1:w719, 2:w692) -> (0:w722:dbl)
      n321 = Power Of X(1:w725, 2:w674) -> (0:w723:dbl)
      n322 = Power Of X(1:w786, 2:w756) -> (0:w773:dbl)
      n323 = Power Of X(1:w786, 2:w754) -> (0:w779:dbl)
      n324 = Power Of X(1:w786, 2:w753) -> (0:w781:dbl)
      n325 = Power Of X(1:w780, 2:w754) -> (0:w785:dbl)
      n326 = Power Of X(1:w780, 2:w756) -> (0:w774:dbl)
      n327 = Power Of X(1:w780, 2:w734) -> (0:w782:dbl)
      n328 = Power Of X(1:w780, 2:w753) -> (0:w783:dbl)
      n329 = Power Of X(1:w786, 2:w734) -> (0:w784:dbl)
      n330 = Compound Arithmetic op=MULTIPLY(w644, w643, 2.69269) -> (w639:dbl)
      n331 = Compound Arithmetic op=MULTIPLY(w645, w646, 2.48243) -> (w641:dbl)
      n332 = Compound Arithmetic op=MULTIPLY(w650, w649, 0.07842) -> (w640:dbl)
      n333 = Compound Arithmetic op=MULTIPLY(w647, w648, 4.47163) -> (w642:dbl)
      n334 = Compound Arithmetic op=MULTIPLY(w583, w582, 2.69269) -> (w578:dbl)
      n335 = Compound Arithmetic op=MULTIPLY(w584, w585, 2.48243) -> (w580:dbl)
      n336 = Compound Arithmetic op=MULTIPLY(w589, w588, 0.07842) -> (w579:dbl)
      n337 = Compound Arithmetic op=MULTIPLY(w586, w587, 4.47163) -> (w581:dbl)
      n338 = Compound Arithmetic op=MULTIPLY(w719, w718, 2.69269) -> (w714:dbl)
      n339 = Compound Arithmetic op=MULTIPLY(w720, w721, 2.48243) -> (w716:dbl)
      n340 = Compound Arithmetic op=MULTIPLY(w725, w724, 0.07842) -> (w715:dbl)
      n341 = Compound Arithmetic op=MULTIPLY(w722, w723, 4.47163) -> (w717:dbl)
      n342 = Compound Arithmetic op=MULTIPLY(w780, w779, 2.69269) -> (w775:dbl)
      n343 = Compound Arithmetic op=MULTIPLY(w781, w782, 2.48243) -> (w777:dbl)
      n344 = Compound Arithmetic op=MULTIPLY(w786, w785, 0.07842) -> (w776:dbl)
      n345 = Compound Arithmetic op=MULTIPLY(w783, w784, 4.47163) -> (w778:dbl)
      n346 = Compound Arithmetic op=unknown(w637, w639, w641, w640, w638, w642) -> (w599:dbl)
      n347 = Compound Arithmetic op=unknown(w576, w578, w580, w579, w577, w581) -> (w539:dbl)
      n348 = Compound Arithmetic op=unknown(w712, w714, w716, w715, w713, w717) -> (w675:dbl)
      n349 = Compound Arithmetic op=unknown(w773, w775, w777, w776, w774, w778) -> (w735:dbl)
      n350 = Power Of X(1:2.718281828459045, 2:w611) -> (0:w609:dbl)
      n351 = Power Of X(1:w599, 2:0.2) -> (0:w652:dbl)
      n352 = Power Of X(1:w539, 2:0.2) -> (0:w591:dbl)
      n353 = Power Of X(1:w675, 2:0.2) -> (0:w727:dbl)
      n354 = Power Of X(1:w735, 2:0.2) -> (0:w788:dbl)
      n355 = Power Of X(1:2.718281828459045, 2:w550) -> (0:w548:dbl)
      n356 = Divide(x=w644, y=w652) -> (x/y=w636:dbl)
      n357 = Divide(x=w583, y=w591) -> (x/y=w575:dbl)
      n358 = Divide(x=w719, y=w727) -> (x/y=w711:dbl)
      n359 = Divide(x=w780, y=w788) -> (x/y=w772:dbl)
      n360 = Power Of X(1:2.718281828459045, 2:w686) -> (0:w684:dbl)
      n361 = Power Of X(1:2.718281828459045, 2:w747) -> (0:w745:dbl)
      n362 = Square(x=w636) -> (x^2=w630:dbl)
      n363 = Square(x=w575) -> (x^2=w569:dbl)
      n364 = Square(x=w711) -> (x^2=w705:dbl)
      n365 = Square(x=w772) -> (x^2=w766:dbl)
      n366 = Power Of X(1:w636, 2:3) -> (0:w629:dbl)
      n367 = Power Of X(1:w575, 2:3) -> (0:w568:dbl)
      n368 = Power Of X(1:w711, 2:3) -> (0:w704:dbl)
      n369 = Power Of X(1:w772, 2:3) -> (0:w765:dbl)
      n370 = Multiply(x=1.36603, y=w636) -> (x*y=w651:dbl)
      n371 = Multiply(x=1.36603, y=w575) -> (x*y=w590:dbl)
      n372 = Multiply(x=1.36603, y=w711) -> (x*y=w726:dbl)
      n373 = Multiply(x=1.36603, y=w772) -> (x*y=w787:dbl)
      n374 = Multiply(x=w629, y=0.11116) -> (x*y=w628:dbl)
      n375 = Multiply(x=w630, y=-0.47719) -> (x*y=w627:dbl)
      n376 = Multiply(x=w568, y=0.11116) -> (x*y=w567:dbl)
      n377 = Multiply(x=w569, y=-0.47719) -> (x*y=w566:dbl)
      n378 = Multiply(x=w704, y=0.11116) -> (x*y=w703:dbl)
      n379 = Multiply(x=w705, y=-0.47719) -> (x*y=w702:dbl)
      n380 = Multiply(x=w765, y=0.11116) -> (x*y=w764:dbl)
      n381 = Multiply(x=w766, y=-0.47719) -> (x*y=w763:dbl)
      n382 = Compound Arithmetic op=unknown(w628, w627, w651) -> (w603:dbl)
      n383 = Compound Arithmetic op=unknown(w567, w566, w590) -> (w543:dbl)
      n384 = Compound Arithmetic op=unknown(w703, w702, w726) -> (w679:dbl)
      n385 = Compound Arithmetic op=unknown(w764, w763, w787) -> (w739:dbl)
      n386 = Subtract(x=w597, y=w603) -> (x-y=w600:dbl)
      n387 = Multiply(x=w603, y=w605) -> (x*y=w604:dbl)
      n388 = Subtract(x=w537, y=w543) -> (x-y=w540:dbl)
      n389 = Multiply(x=w543, y=w532) -> (x*y=w544:dbl)
      n390 = Subtract(x=w673, y=w679) -> (x-y=w676:dbl)
      n391 = Multiply(x=w679, y=w668) -> (x*y=w680:dbl)
      n392 = Subtract(x=w733, y=w739) -> (x-y=w736:dbl)
      n393 = Multiply(x=w739, y=w741) -> (x*y=w740:dbl)
      n394 = Multiply(x=w609, y=w600) -> (x*y=w601:dbl)
      n395 = Multiply(x=w548, y=w540) -> (x*y=w541:dbl)
      n396 = Multiply(x=w684, y=w676) -> (x*y=w677:dbl)
      n397 = Multiply(x=w745, y=w736) -> (x*y=w737:dbl)
      n398 = Add(x=w601, y=w604) -> (x+y=w596:dbl)
      n399 = Add(x=w541, y=w544) -> (x+y=w536:dbl)
      n400 = Add(x=w677, y=w680) -> (x+y=w672:dbl)
      n401 = Add(x=w737, y=w740) -> (x+y=w732:dbl)
      n402 = Multiply(x=w596, y=w516) -> (x*y=w595:dbl)
      n403 = Multiply(x=w536, y=w516) -> (x*y=w535:dbl)
      n404 = Multiply(x=w672, y=w660) -> (x*y=w671:dbl)
      n405 = Multiply(x=w732, y=w660) -> (x*y=w731:dbl)
      n406 = Subtract(x=w597, y=w595) -> (x-y=w529:dbl)
      n407 = Subtract(x=w537, y=w535) -> (x-y=w528:dbl)
      n408 = Subtract(x=w673, y=w671) -> (x-y=w663:dbl)
      n409 = Subtract(x=w733, y=w731) -> (x-y=w664:dbl)
      n410 = case shown="False" w531 {
        tunnel: [w808 w814] -> w515
        tunnel: w516 -> [_ w815]
        tunnel: w530 -> [w811 _]
        tunnel: w529 -> [w810 _]
        tunnel: w528 -> [w809 _]
        frame False {
          n411 = case shown="False" w811 {
            tunnel: [w812 w813] -> w808
            tunnel: w810 -> [_ w813]
            tunnel: w809 -> [w812 _]
            frame False {
            }
            frame True {
            }
          }
        }
        frame True {
          n412 = Subtract(x=1.0, y=w815) -> (x-y=w814:dbl)
        }
      }
      n413 = case shown="False" w667 {
        tunnel: [w817 w823] -> w666
        tunnel: w660 -> [_ w824]
        tunnel: w665 -> [w820 _]
        tunnel: w664 -> [w819 _]
        tunnel: w663 -> [w818 _]
        frame False {
          n414 = case shown="False" w820 {
            tunnel: [w821 w822] -> w817
            tunnel: w819 -> [_ w822]
            tunnel: w818 -> [w821 _]
            frame False {
            }
            frame True {
            }
          }
        }
        frame True {
          n415 = Subtract(x=1.0, y=w824) -> (x-y=w823:dbl)
        }
      }
      n416 = Multiply(x=w515, y=w497) -> (x*y=w498:dbl)
      n417 = Multiply(x=w666, y=w508) -> (x*y=w507:dbl)
      n418 = case shown="False" w501 {
        tunnel: 0.0 -> [w793 w800]
        tunnel: w508 -> [w792 w807]
        tunnel: w507 -> [w791 w806]
        tunnel: "AFP Efficiency" -> [_ w794]
        tunnel: [w791 w802] -> w505
        tunnel: [w792 w801] -> w504
        tunnel: [w793 w800] -> w503
        tunnel: w498 -> [w790 w799]
        tunnel: [w790 w798] -> w499
        tunnel: w497 -> [w789 w797]
        tunnel: [w789 w795] -> w496
        frame False {
        }
        frame True {
          n419 = Negate(x=w797) -> (-x=w796:dbl)
          n420 = Negate(x=w799) -> (-x=w805:dbl)
          n421 = Negate(x=w806) -> (-x=w804:dbl)
          n422 = Negate(x=w807) -> (-x=w803:dbl)
          n423 = Multiply(x=w796, y=w794) -> (x*y=w795:dbl)
          n424 = Multiply(x=w805, y=w794) -> (x*y=w798:dbl)
          n425 = Multiply(x=w804, y=w794) -> (x*y=w802:dbl)
          n426 = Multiply(x=w803, y=w794) -> (x*y=w801:dbl)
        }
      }
    }
    n427 = Divide(x=12.0, y=500.0) -> (x/y=w102:dbl)
    n428 = Divide(x=12.0, y=500.0) -> (x/y=w140:dbl)
    n429 = Divide(x=12.0, y=500.0) -> (x/y=w144:dbl)
    n430 = Divide(x=12.0, y=500.0) -> (x/y=w98:dbl)
    n431 = Multiply(x=w94, y=w102) -> (x*y=→"upper R-value AFP":dbl)
    n432 = Multiply(x=w133, y=w140) -> (x*y=→"lower R-value":dbl)
    n433 = Multiply(x=w136, y=w144) -> (x*y=→"upper R-value":dbl)
    n434 = Multiply(x=w91, y=w98) -> (x*y=→"lower R-value AFP":dbl)
    n435 = case shown="True" w182 {
      tunnel: w186 -> [_ w485]
      tunnel: w85 -> [w481 w484]
      tunnel: w85 -> [_ w483]
      tunnel: [w481 w483] -> w185
      tunnel: [w480 w482] -> w173
      tunnel: w176 -> [w480 _]
      frame False {
      }
      frame True {
        n436 = Subtract(x=w485, y=w484) -> (x-y=w482:dbl[])
      }
    }
    n437 = case shown="True" w182 {
      tunnel: w200 -> [_ w491]
      tunnel: w191 -> [w487 w490]
      tunnel: w199 -> [_ w489]
      tunnel: [w487 w489] -> w183
      tunnel: [w486 w488] -> w172
      tunnel: w176 -> [w486 _]
      frame False {
      }
      frame True {
        n438 = Subtract(x=w491, y=w490) -> (x-y=w488:dbl[])
      }
    }
    n439 = Add(x=w185, y=w78) -> (x+y=w68:dbl[])
    n440 = Add(x=w173, y=w78) -> (x+y=w70:dbl[])
    n441 = Add(x=w79, y=w172) -> (x+y=w72:dbl[])
    n442 = Add(x=w79, y=w183) -> (x+y=w74:dbl[])
    n443 = call "FitAndSubtract.vi"("Array 4"=w65, "Array 3"=w66, "Numeric"=w67, "Array in"=w68) -> ("Array out"=w69:dbl[])  [unwired: 6 in, 1 out]
    n444 = call "FitAndSubtract.vi"("Array 4"=w65, "Array 3"=w66, "Numeric"=w67, "Array in"=w70) -> ("Array out"=w71:dbl[])  [unwired: 6 in, 1 out]
    n445 = call "FitAndSubtract.vi"("Array 4"=w65, "Array 3"=w66, "Numeric"=w67, "Array in"=w72) -> ("Array out"=w75:dbl[])  [unwired: 6 in, 1 out]
    n446 = Bundle(w66, w74) -> (w225:cluster{dbl[], dbl[]})  [unwired: 1 in]
    n447 = call "FitAndSubtract.vi"("Array 4"=w65, "Array 3"=w66, "Numeric"=w67, "Array in"=w74) -> ("Best Polynomial Fit"=w73:dbl[], "Array out"=w76:dbl[])  [unwired: 6 in]
    n448 = Bundle(w66, "Best Polynomial Fit"=w73) -> (w159:cluster{dbl[], "Best Polynomial Fit":dbl[]})  [unwired: 1 in]
    n449 = call "rhozero.vi"("Array in"=w69) -> ("Array out"=w180:dbl[])  [unwired: 10 in]
    n450 = call "rhominus.vi"("Array"=w76, "Array 2"=w69) -> ("Array 3"=w179:dbl[])  [unwired: 9 in]
    n451 = Add(x=w75, y=w71) -> (x+y=w174:dbl[])
    n452 = Subtract(x=w75, y=w71) -> (x-y=w175:dbl[])
    n453 = call "rhoplus.vi"("Array 3"=w69, "Array in"=w76) -> ("Array out"=w181:dbl[])  [unwired: 9 in]
    n454 = Build Array(w225, w159) -> (→"Signal and Fit (P)":cluster{dbl[], "Best Polynomial Fit":dbl[]}[])
    n455 = Divide(x=w174, y=w171) -> (x/y=w170:dbl[])
    n456 = Subtract(x=w181, y=w180) -> (x-y=w168:dbl[])
    n457 = Divide(x=w175, y=w171) -> (x/y=w169:dbl[])
    n458 = Bundle(w66, "Array out"=w180) -> ()  [unwired: 1 in, 1 out]
    n459 = Bundle(w66, "Array out"=w181) -> ()  [unwired: 1 in, 1 out]
    n460 = Subtract(x=w180, y=w179) -> (x-y=w167:dbl[])
    n461 = Bundle(w66, "Array 3"=w179) -> ()  [unwired: 1 in, 1 out]
    n462 = Reverse 1D Array(array=w170) -> (reversed array=w178:dbl[])
    n463 = Reverse 1D Array(array=w169) -> (reversed array=w177:dbl[])
    n464 = Divide(x=w178, y=w171) -> (x/y=w82:dbl[])
    n465 = Divide(x=w177, y=w171) -> (x/y=w83:dbl[])
    n466 = Add(x=w167, y=w82) -> (x+y=w165:dbl[])
    n467 = Add(x=w168, y=w83) -> (x+y=w166:dbl[])
    n468 = Subtract(x=w166, y=w165) -> (x-y=w153:dbl[])
    n469 = Add(x=w165, y=w166) -> (x+y=w60:dbl[])
    n470 = Bundle(w66, w166) -> (w160:cluster{dbl[], dbl[]})  [unwired: 1 in]
    n471 = Bundle(w66, w165) -> (w161:cluster{dbl[], dbl[]})  [unwired: 1 in]
    n472 = Add Array Elements(numeric array=w60) -> (sum=w155:dbl)
    n473 = Add Array Elements(numeric array=w153) -> (sum=w154:dbl)
    n474 = Bundle(w66, w153) -> (→"Corrected Data (Q)":cluster{dbl[], dbl[]})  [unwired: 1 in]
    n475 = Bundle(w66, w60) -> (w162:cluster{dbl[], dbl[]})  [unwired: 1 in]
    n476 = Array To Spreadsheet String(delimiter (Tab)=",", array=w60, 3:"%f") -> (spreadsheet string=w64:string)
    n477 = Format Into String(format string="%d", initial string="", w53) -> (resulting string=w115:string)  [unwired: 1 in, 1 out]
    n478 = Build Array(w162, w160, w161) -> (→"Corrected Data (P)":cluster{dbl[], dbl[]}[])
    n479 = Number To Fractional String(number="Saturation\nPolarization", precision (6)=i16 2) -> (F-format string=w62:string)  [unwired: 2 in]
    n480 = Divide(x=12.0, y=500.0) -> (x/y=w151:dbl)
    n481 = Divide(x=12.0, y=500.0) -> (x/y=w145:dbl)
    n482 = Multiply(x=w155, y=w151) -> (x*y=w152:dbl)
    n483 = Multiply(x=w154, y=w145) -> (x*y=w148:dbl)
    n484 = Absolute Value(x=w152) -> (abs(x)=w105:dbl)
    "Reimann\nsum of P" <- w105
    n485 = Concatenate Strings(w115, ",", w62, ",", w64) -> (w112:string)
    n486 = Absolute Value(x=w148) -> (abs(x)=w132:dbl)
    "Reimann \nsum of Q" <- w132
    n487 = Write to Text File(file (use dialog)=w121, text=w112, error in=w120) -> (refnum out=w119:refnum<file>, error out=w118:errorcluster)  [unwired: 1 in, 1 out]
    n488 = Square(x=w105) -> (x^2=w103:dbl)
    n489 = Bundle(w105, w132) -> (→"Total Polarization (P)":cluster{dbl, dbl})  [unwired: 1 in]
    n490 = Quotient & Remainder(x=w53, y="Batch Size") -> (x-y*floor(x/y)=w51:i32)  [unwired: 1 out]
    n491 = Multiply(x=3, y=w103) -> (x*y=w107:dbl)
    n492 = Equal To 0?(x=w51) -> (x = 0?=w50:bool)
    n493 = Select(t="Training?", s=w50, f=FALSE) -> (s? t:f=w47:bool)
    n494 = call "Ann_int.vi"("Data"=w60, "Loss Function"="Loss Function", "Regularization"="Regularization", "Target"="Saturation\nPolarization", "Training?"=w47, "Parameters"=w58, "Adam Data In"=w54) -> ("Output"=→"NN Output":dbl, "Error"=w44:dbl, "Adjusted Parameters"=w42:T4, "Adam Data Out"=w55:T2)  [unwired: 5 in]
    "NN Error" <- w44
    "NN Loss" <- w44
    n495 = Subtract(x=4, y=w107) -> (x-y=w104:dbl)
    n496 = Square Root(x=w104) -> (sqrt(x)=w109:dbl)
    n497 = Less?(x=w45, y=w44) -> (x < y?=w43:bool)
    n498 = Subtract(x=2, y=w109) -> ()  [unwired: 1 out]
    n499 = Select(t=w45, s=w43, f=w44) -> (s? t:f=w46:dbl)
    n500 = Select(t=w40, s=w43, f=w42) -> (s? t:f=w41:T4)
  }
  n501 = invoke class="VI" method="Default Vals.Reinit All"(reference=w38) -> ()  [unwired: 2 in, 3 out]
  n502 = property on="Total Polarization (P)" class="WFChart (strict)"("History Data"=cluster{dbl, dbl}[] []) -> ()  [unwired: 2 in, 2 out]
  n503 = property on="NN Training Loss" class="WFChart (strict)"("History Data"=dbl[] []) -> ()  [unwired: 2 in, 2 out]
  n504 = Close File(refnum=w34, error in=w33) -> ()  [unwired: 2 out]
  n505 = Flatten To XML(6:w2) -> (2:w30:string)
  n506 = call-poly <vilib>:"Write to XML File.vi"("XML Input"=w30, "XML File Path"="Parameters File Path") -> ()  [unwired: 7 in, 3 out]
